vi "TCP Server - Parse first message.vi"(8 "error in (no error)":errorcluster, 9 "Message":string, 10 "TCP Client ID":refnum<k5>, 11 "TCP Server in":refnum<class "TCP Server.lvclass">) -> (0 "error out":errorcluster, 1 "External error out":errorcluster, 3 "TCP Server out":refnum<class "TCP Server.lvclass">)   [LabVIEW 2020, in "TALOS.lvlib" / "TCP Server.lvlib" / "TCP Server.lvclass"]
uses:
  TCP Server.lvclass
  TCP Server Msg Actions.ctl
  Ancestor/Ancestor/Ancestor.lvclass/Ancestor.ctl
  FGV/Error Memory/Get Error Description.vi
  Ancestor/Ancestor/Read ID.vi
  Support VIs/Get Class Name.vi
  <vilib>/Utility/error.llb/Clear Errors.vi
  FGV/Error Memory/Error Memory Core.vi
  <vilib>/AdvancedString/Delimited String to 1D String Array.vi
  Support VIs/Circus Root Path.vi
  FGV/Error Memory/Error Crt Lvl checker.vi
  FGV/Error Memory/Error Memory Core.vi/40c8088d-b597-4017-91af-faa98e00292e.vi
  FGV/Error Memory/Error Memory Core.vi/d4a3ab98-063c-4e44-b43d-fbdcfe6c2be2.vi
  Support VIs/Global Constants.vi
  Support VIs/Global Memory.vi
  <userlib>/_OpenG.lib/string/string.llb/Trim Whitespace (String)__ogtk.vi
  <vilib>/Utility/LVClass/Get LV Class Name.vi
  Support VIs/Is in Packed Library.vi
  Support VIs/TALOS Root path.vi
  Support VIs/Read CSV worksheet.vi
  <vilib>/Utility/error.llb/General Error Handler.vi
  Support VIs/Error Log.vi
  Ancestor/Ancestor/Ancestor.lvclass
  <vilib>/Comparison/Equal/Equal Functor/Equal Functor.lvclass
  TALOS.lvlib
  bd90c6b7-bc86-460d-9dd7-41153e43b143.vi
  <userlib>/_OpenG.lib/string/string.llb/openg_string.lvlib
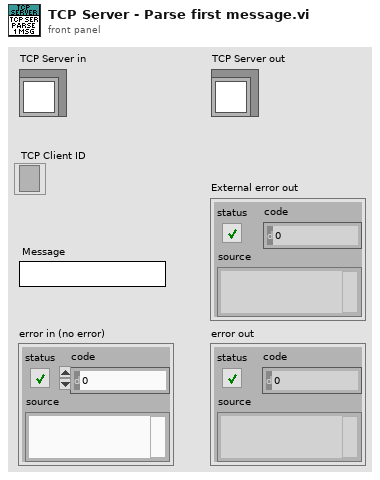
[diagram p1: front panel]
types:
  T1 = typedef "TALOS.lvlib/TCP Server.lvlib/TCP Server.lvclass/TCP Server Msg Actions.ctl" = enum16{"Spawn TCP Listener/Writer", "External Error", "I Exist", "Who the hell is this guy?", "Do nothing"}
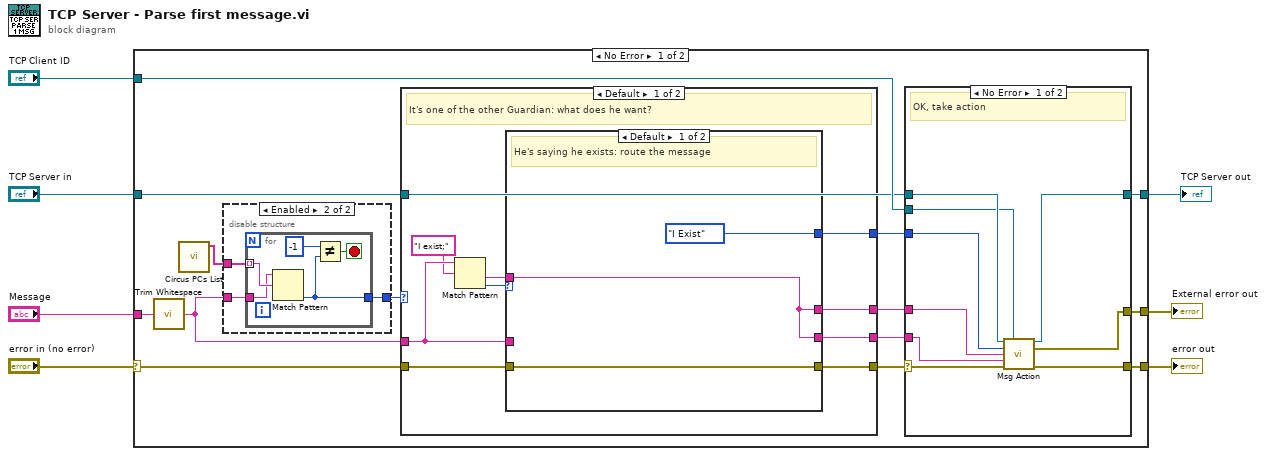
[diagram p0: block diagram]
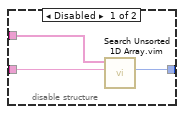
[diagram p2: hidden frame]
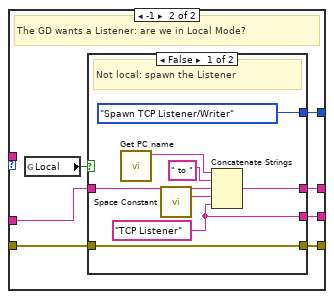
[diagram p3: hidden frame]
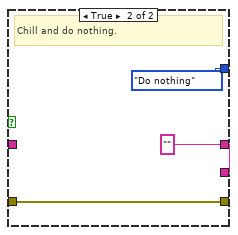
[diagram p4: hidden frame]
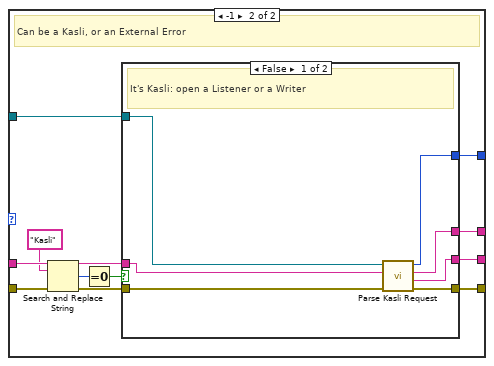
[diagram p5: hidden frame]
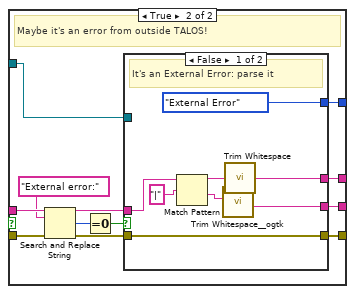
[diagram p6: hidden frame]
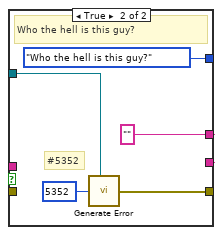
[diagram p7: hidden frame]
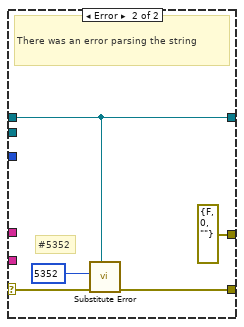
[diagram p8: hidden frame]
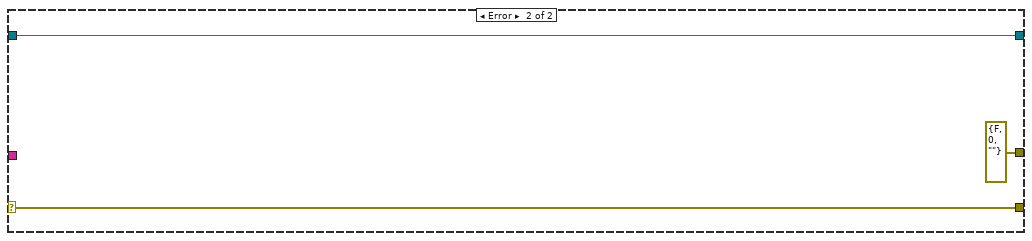
[diagram p9: hidden frame]
diagram:
  n1 = case shown="No Error" "error in (no error)" {
    selector: "error in (no error)" -> [w21 w122]
    tunnel: "Message" -> [w17 _]
    tunnel: "TCP Client ID" -> [w16 _]
    tunnel: [w15 w122] -> w4
    tunnel: "TCP Server in" -> [w14 w123]
    tunnel: [w10 w123] -> w2
    tunnel: [w8 errorcluster {"status"=FALSE, "code"=0, "source"=""} ("error out")] -> w1
    frame No Error {
      n2 = call <vilib>:"Trim Whitespace.vi"("string"=w17) -> ("trimmed string"=w20:string)  [unwired: 1 in]
      n3 = call "Circus PCs List.vi"() -> ("PC List out"=w18:string[])  [unwired: 10 in, 1 out]
      n4 = disable-structure shown="Enabled" {
        disable-tunnel: w20 -> [w24 w27]
        disable-tunnel: [w23 w25] -> w19
        disable-tunnel: w18 -> [w22 w26]
        frame Disabled {
          n5 = call "Search Unsorted 1D Array.vim"("element"=w24, "unsorted 1D array"=w22) -> ("index of element"=w23:i32)  [unwired: 9 in]
        }
        frame Enabled {
          n6 = for {
            tunnel: w27 -> [w31]
            tunnel: w26 -> [w32] mode=indexing
            tunnel: [w29] -> w25
            stop <- w30 stop-if-true
            n7 = Match Pattern(string=w31, regular expression=w32) -> (offset past match=w29:i32)  [unwired: 1 in, 3 out]
            n8 = Not Equal?(x=-1, y=w29) -> (x != y?=w30:bool)
          }
        }
      }
      n9 = case shown="Default" w19 {
        tunnel: [w41 w69] -> w13
        tunnel: w20 -> [w37 w73]
        tunnel: w21 -> [w40 w68]
        tunnel: [w39 w66] -> w12
        tunnel: w14 -> [_ w65]
        tunnel: [w38 w64] -> w11
        tunnel: [w35 w63] -> w9
        frame Default {
          # "It's one of the other Guardian: what does he want?"
          n10 = Match Pattern(string=w37, regular expression="I exist;") -> (after substring=w33:string, offset past match=w34:i32)  [unwired: 1 in, 2 out]
          n11 = case shown="Default" w34 {
            tunnel: [w44 w51] -> w41
            tunnel: w37 -> [_ w50]
            tunnel: w40 -> [w44 w49]
            tunnel: [w42 w48] -> w39
            tunnel: [w42 w46] -> w38
            tunnel: [TCP_Server_Msg_Actions."I Exist" w45] -> w35
            tunnel: w33 -> [w42 _]
            frame Default {
              # "He's saying he exists: route the message"
            }
            frame -1 {
              # "The GD wants a Listener: are we in Local Mode?"
              n12 = global read "Global Constants.vi" "Local"() -> (w47:bool)
              n13 = case shown="False" w47 {
                tunnel: [w53 w62] -> w51
                tunnel: w50 -> [w57 _]
                tunnel: w49 -> [w53 w62]
                tunnel: [w55 w61] -> w48
                tunnel: [w54 w61] -> w46
                tunnel: [TCP_Server_Msg_Actions."Spawn TCP Listener/Writer" TCP_Server_Msg_Actions."Do nothing"] -> w45
                frame False {
                  w54 = "TCP Listener" ("uService Class Name")
                  # "Not local: spawn the Listener"
                  n14 = call "Get PC name.vi"() -> ("Hostname"=w59:string)  [unwired: 10 in, 1 out]
                  n15 = call <vilib>:"Space Constant.vi"() -> ("String"=w56:string)
                  n16 = Concatenate Strings(w59, " to " ("string"), w57, w56, w54) -> (w55:string)
                }
                frame True {
                  w61 = ""
                  # "Chill and do nothing."
                }
              }
            }
          }
        }
        frame -1 {
          # "Can be a Kasli, or an External Error"
          n17 = Search and Replace String(input string=w73, search string="Kasli", error in=w68) -> (result string=w74:string, number of replacements=w71:i32, error out=w67:errorcluster)  [unwired: 5 in, 1 out]
          n18 = Equal To 0?(x=w71) -> (x = 0?=w70:bool)
          n19 = case shown="False" w70 {
            tunnel: [w80 w93] -> w69
            tunnel: w67 -> [w76 w87]
            tunnel: w74 -> [w77 w89]
            tunnel: [w78 w91] -> w66
            tunnel: w65 -> [w79 w92]
            tunnel: [w81 w86] -> w64
            tunnel: [w75 w82] -> w63
            frame False {
              # "It's Kasli: open a Listener or a Writer"
              n20 = call "Parse Kasli Request.vi"("error in (no error)"=w76, "Message part"=w77, "TCP Server in"=w79) -> ("error out"=w80:errorcluster, "uService Class Name"=w81:string, "uService ID"=w78:string, "TCP Server Msg Actions"=w75:T1)  [unwired: 5 in]
            }
            frame True {
              # "Maybe it's an error from outside TALOS!"
              n21 = Search and Replace String(input string=w89, search string="External error:", error in=w87) -> (result string=w84:string, number of replacements=w90:i32, error out=w83:errorcluster)  [unwired: 5 in, 1 out]
              n22 = Equal To 0?(x=w90) -> (x = 0?=w85:bool)
              n23 = case shown="False" w85 {
                tunnel: [w101 w105] -> w93
                tunnel: w92 -> [_ w104]
                tunnel: [w95 w103] -> w91
                tunnel: [w97 w103] -> w86
                tunnel: w84 -> [w99 _]
                tunnel: w83 -> [w101 _]
                tunnel: [TCP_Server_Msg_Actions."External Error" TCP_Server_Msg_Actions."Who the hell is this guy?"] -> w82
                frame False {
                  # "It's an External Error: parse it"
                  n24 = Match Pattern(string=w99, regular expression="|") -> (before substring=w96:string, after substring=w98:string)  [unwired: 1 in, 2 out]
                  n25 = call-poly <userlib>:"Trim Whitespace__ogtk.vi"("String in"=w98) -> ("String out"=w97:string)  [unwired: 6 in]
                  n26 = call <vilib>:"Trim Whitespace.vi"("string"=w96) -> ("trimmed string"=w95:string)  [unwired: 1 in]
                }
                frame True {
                  w103 = "" ("uService ID")
                  # "#5352"
                  # "Who the hell is this guy?"
                  n27 = call "Generate Error.vi"("Class"=w104, "Error Code"=5352) -> ("error out"=w105:errorcluster)  [unwired: 5 in]
                }
              }
            }
          }
        }
      }
      n28 = case shown="No Error" w13 {
        selector: w13 -> [w114 w120]
        tunnel: w16 -> [w110 _]
        tunnel: [w115 w119] -> w15
        tunnel: w14 -> [w111 w117]
        tunnel: w12 -> [w108 _]
        tunnel: w11 -> [w107 _]
        tunnel: [w113 w117] -> w10
        tunnel: w9 -> [w109 _]
        tunnel: [w112 errorcluster {"status"=FALSE, "code"=0, "source"=""} ("error out")] -> w8
        frame No Error {
          # "OK, take action"
          n29 = call "Msg Action.vi"("TCP Server in"=w111, "TCP Client ID"=w110, "TCP Server Msg Actions"=w109, "uService ID"=w108, "uService Class Name"=w107, "error in (no error)"=w114) -> ("TCP Server out"=w113:refnum<class "TCP Server.lvclass">, "External Error out"=w112:errorcluster, "error out"=w115:errorcluster)  [unwired: 7 in]
        }
        frame Error {
          # "#5352"
          # "There was an error parsing the string"
          n30 = call "Substitute Error.vi"("LabVIEW Object"=w117, "error in (no error)"=w120, "Error Code"=5352) -> ("error out"=w119:errorcluster)  [unwired: 8 in]
        }
      }
    }
    frame Error {
    }
  }
  "error out" <- w4
  "TCP Server out" <- w2
  "External error out" <- w1
